vi "Axis.vi"   [LabVIEW 2021]
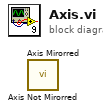
[diagram p0: block diagram]
diagram:
  n1 = call "Axis Not Mirorred.vi"() -> ()  [unwired: 10 in, 2 out]
  n2 = call "Axis Mirorred.vi"() -> ()  [unwired: 10 in, 2 out]
